vi "Encoder Sim Data.vi"(10 "Encoder in":i32) -> (2 "Encoder out":i32)   [LabVIEW 2014, in "SimSyA.lvlib"]
uses:
  SimSyA.lvlib
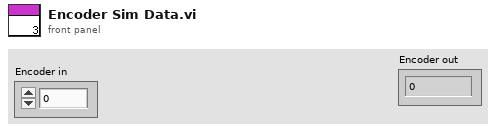
[diagram p1: front panel]
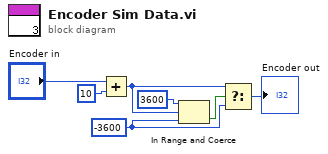
[diagram p0: block diagram]
diagram:
  w2 = -3600 ("lower limit")
  n1 = Add(x="Encoder in", y=10) -> (x+y=w3:i32)
  n2 = In Range and Coerce(upper limit=3600, x=w3, lower limit=w2) -> (In Range?=w4:bool)  [unwired: 1 out]
  n3 = Select(t=w3, s=w4, f=w2) -> (s? t:f=→"Encoder out":i32)
